vi "Append unique suffix.vi"(6 "Extention":string, 7 "Suffix":string, 8 "error in (no error)":errorcluster, 10 "ovewrite ?":bool, 11 "Path":path) -> (0 "error out":errorcluster, 3 "Path out":path)   [LabVIEW 2021]
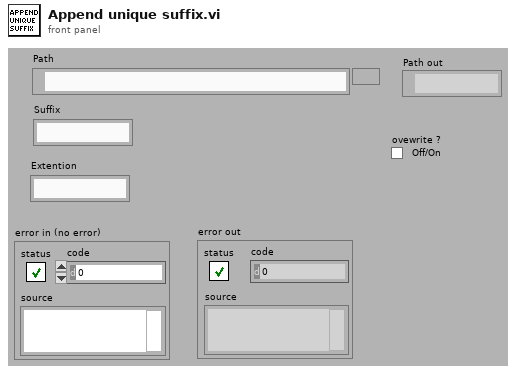
[diagram p1: front panel]
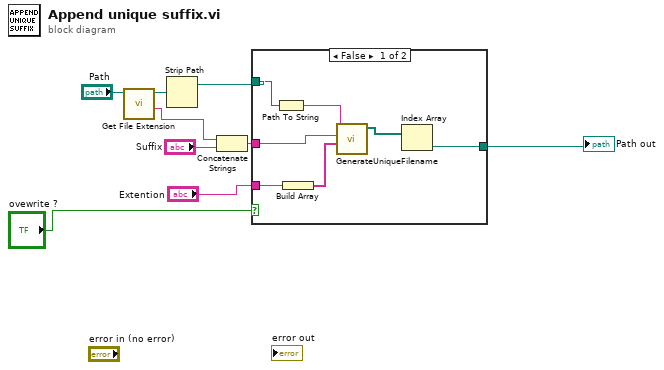
[diagram p0: block diagram]
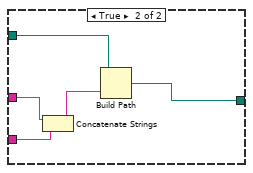
[diagram p2: hidden frame]
diagram:
  n1 = call <vilib>:"Get File Extension.vi"("file"="Path") -> ("filename without extension"=w4:string, "dup file"=w3:path)  [unwired: 6 in, 3 out]
  n2 = Strip Path(path=w3) -> (stripped path=w6:path)  [unwired: 1 out]
  n3 = Concatenate Strings(w4, "Suffix") -> (w8:string)
  n4 = case shown="False" "ovewrite ?" {
    tunnel: w8 -> [w16 w21]
    tunnel: "Extention" -> [w15 w20]
    tunnel: w6 -> [w11 w19]
    tunnel: [w12 w17] -> w2
    frame False {
      n5 = Path To String(path=w11) -> (string=w10:string)
      n6 = Build Array(w15) -> (w14:string[])
      n7 = call "GenerateUniqueFilename.vi"("File Name Suffixes"=w14, "File Name Prefix"=w16, "Folder"=w10) -> ("Paths"=w13:path[])  [unwired: 7 in, 1 out]
      n8 = Index Array(array=w13) -> (element=w12:path)  [unwired: 1 in]
    }
    frame True {
      n9 = Concatenate Strings(w21, w20) -> (w18:string)
      n10 = Build Path(base path=w19, name or relative path=w18) -> (appended path=w17:path)
    }
  }
  "Path out" <- w2
